vi "Acme Subtract.vi"(8 "error in (no error)":errorcluster, 10 "y":dbl, 11 "x":dbl) -> (0 "error out":errorcluster, 3 "difference":dbl)   [LabVIEW 2014, in "acme_math.lvlib"]
doc: "Subtract two numbers."
uses:
  acme_math.lvlib
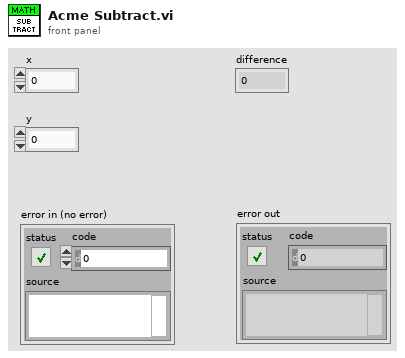
[diagram p1: front panel]
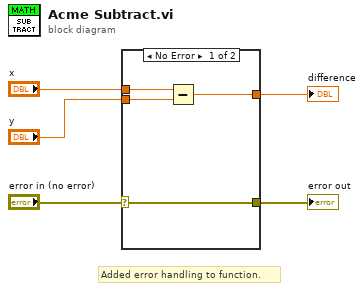
[diagram p0: block diagram]
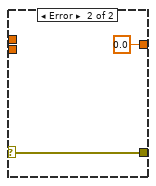
[diagram p2: hidden frame]
diagram:
  # "Added error handling to function."
  n1 = case shown="No Error" "error in (no error)" {
    selector: "error in (no error)" -> [w6 w11]
    tunnel: "y" -> [w9 _]
    tunnel: "x" -> [w8 _]
    tunnel: [w7 0.0] -> w3
    tunnel: [w6 w11] -> w1
    frame No Error {
      n2 = Subtract(x=w8, y=w9) -> (x-y=w7:dbl)
    }
    frame Error {
    }
  }
  "difference" <- w3
  "error out" <- w1
